vi "Draw Feature Position.vi"(6 "Color":u32(colorbox)=65280, 8 "Error In":errorcluster, 10 "Feature Ponts":cluster{"X":sgl, "Y":sgl}[](array[cluster]), 11 "Image":T1) -> (0 "Error Out":errorcluster, 3 "Image Out":T1)   [LabVIEW 2012]
uses:
  <vilib>/vision/Image Controls.llb/IMAQ Image.ctl
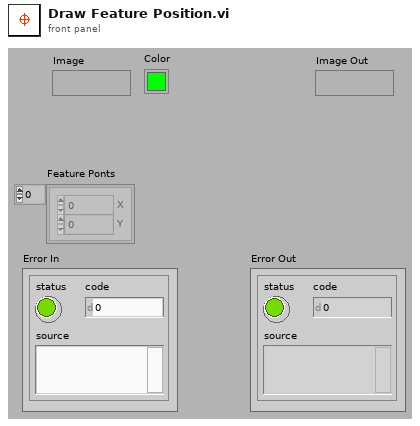
[diagram p1: front panel]
types:
  T1 = typedef "IMAQ Image.ctl" = refnum<image>
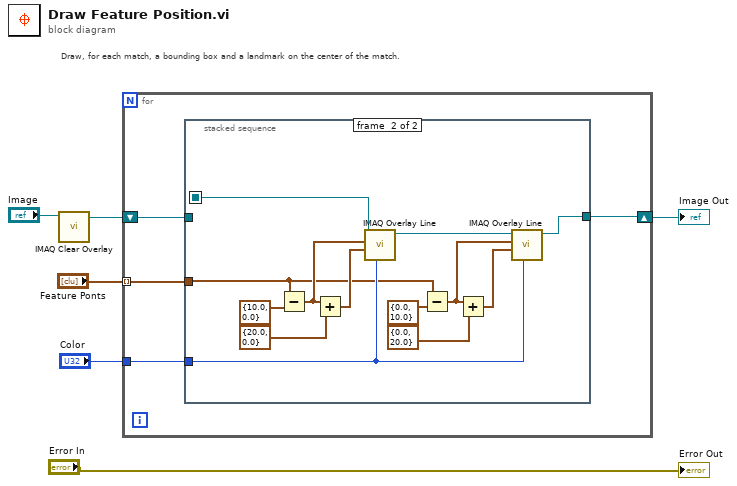
[diagram p0: block diagram]
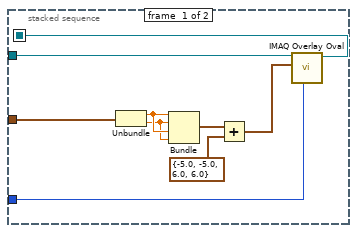
[diagram p2: hidden frame]
diagram:
  # "Draw, for each match, a bounding box and a landmark on the center of the match."
  n1 = call "IMAQ Clear Overlay"("Image"="Image") -> ("Image Out"=w4:T1)  [unwired: 2 in, 8 out]
  n2 = for {
    shift-right: [w8] -> w5
    shift-left: w4 -> [w10]
    tunnel: "Feature Ponts" -> [w7] mode=indexing
    tunnel: "Color" -> [w9]
    n3 = stacked-sequence {
      seq-local: [w18 _] -> [_ w20]
      tunnel: w7 -> [w11 w22]
      tunnel: w10 -> [w19 _]
      tunnel: w9 -> [w17 w24]
      tunnel: [_ w21] -> w8
      frame #0 {
        n4 = Unbundle(w11) -> ("X"=w16:sgl, "Y"=w15:sgl)
        n5 = Bundle("X"=w16, "Y"=w15, "X"=w16, "Y"=w15) -> (w14:cluster{"X":sgl, "Y":sgl, "X":sgl, "Y":sgl})  [unwired: 1 out]
        n6 = Add(x=w14, y=cluster{"y":sgl, "x":sgl, "y":sgl, "x":sgl} {"y"=-5.0, "x"=-5.0, "y"=6.0, "x"=6.0}) -> (x+y=w12:cluster{sgl, sgl, sgl, sgl})
        n7 = call "IMAQ Overlay Oval"("Color"=w17, "Bounding Rectangle"=w12, "Image"=w19) -> ("Image Out"=w18:T1)  [unwired: 3 in, 5 out]
      }
      frame #1 {
        n8 = Subtract(x=w22, y=cluster{"x":sgl, "y":sgl} {"x"=10.0, "y"=0.0}) -> (x-y=w31:cluster{sgl, sgl})
        n9 = Add(x=w31, y=cluster{"x":sgl, "y":sgl} {"x"=20.0, "y"=0.0}) -> (x+y=w29:cluster{sgl, sgl})
        n10 = call "IMAQ Overlay Line"("Color"=w24, "End Point"=w29, "Start Point"=w31, "Image"=w20) -> ("Image Out"=w23:T1)  [unwired: 2 in, 5 out]
        n11 = Subtract(x=w22, y=cluster{"x":sgl, "y":sgl} {"x"=0.0, "y"=10.0}) -> (x-y=w27:cluster{sgl, sgl})
        n12 = Add(x=w27, y=cluster{"x":sgl, "y":sgl} {"x"=0.0, "y"=20.0}) -> (x+y=w28:cluster{sgl, sgl})
        n13 = call "IMAQ Overlay Line"("Color"=w24, "End Point"=w28, "Start Point"=w27, "Image"=w23) -> ("Image Out"=w21:T1)  [unwired: 2 in, 5 out]
      }
    }
  }
  "Image Out" <- w5
  "Error Out" <- "Error In"
